vi "Known Targets.vi"() -> (3 "targets        project targetItem name              menu to use                    fpga sub                                           suffix info":T1(array[cluster])=[{"name"="My Computer", "owner"=TRUE, "none"=FALSE, "one"=FALSE, "auto"=FALSE, "choose"=FALSE, "opt#"=FALSE, "ipaddr"=FALSE, "[loc,]mod"=FALSE, "TSname"=""}, {"name"="Networked Computer/Device", "owner"=FALSE, "none"=TRUE, "one"=FALSE, "auto"=FALSE, "choose"=FALSE, "opt#"=TRUE, "ipaddr"=TRUE, "[loc,]mod"=FALSE, "TSname"="CPU"}, {"name"="RT Desktop Target", "owner"=FALSE, "none"=TRUE, "one"=FALSE, "auto"=FALSE, "choose"=FALSE, "opt#"=TRUE, "ipaddr"=TRUE, "[loc,]mod"=FALSE, "TSname"="RT cpu"}, {"name"="RT ELVIS RIO Target", "owner"=FALSE, "none"=TRUE, "one"=TRUE, "auto"=FALSE, "choose"=FALSE, "opt#"=TRUE, "ipaddr"=TRUE, "[loc,]mod"=FALSE, "TSname"="RT ELVIS"}, {"name"="RT myRIO Target", "owner"=FALSE, "none"=TRUE, "one"=TRUE, "auto"=FALSE, "choose"=FALSE, "opt#"=TRUE, "ipaddr"=TRUE, "[loc,]mod"=FALSE, "TSname"="RT myRIO"}, {"name"="RT CompactRIO Target", "owner"=FALSE, "none"=TRUE, "one"=TRUE, "auto"=FALSE, "choose"=FALSE, "opt#"=TRUE, "ipaddr"=TRUE, "[loc,]mod"=FALSE, "TSname"="RT cRIO"}, {"name"="RT Single-Board RIO Target", "owner"=FALSE, "none"=TRUE, "one"=TRUE, "auto"=FALSE, "choose"=FALSE, "opt#"=TRUE, "ipaddr"=TRUE, "[loc,]mod"=FALSE, "TSname"="RT sbRIO"}, {"name"="RT roboRIO Target", "owner"=FALSE, "none"=TRUE, "one"=TRUE, "auto"=FALSE, "choose"=FALSE, "opt#"=TRUE, "ipaddr"=TRUE, "[loc,]mod"=FALSE, "TSname"="RT roboRIO"}, {"name"="Ethernet RIO Target", "owner"=FALSE, "none"=TRUE, "one"=TRUE, "auto"=FALSE, "choose"=FALSE, "opt#"=TRUE, "ipaddr"=TRUE, "[loc,]mod"=FALSE, "TSname"="RT netRIO"}, {"name"="RT FlexRIO", "owner"=FALSE, "none"=TRUE, "one"=FALSE, "auto"=TRUE, "choose"=FALSE, "opt#"=TRUE, "ipaddr"=TRUE, "[loc,]mod"=FALSE, "TSname"="RT flexRIO"}, {"name"="RT PXI Target", "owner"=FALSE, "none"=FALSE, "one"=FALSE, "auto"=FALSE, "choose"=TRUE, "opt#"=FALSE, "ipaddr"=FALSE, "[loc,]mod"=FALSE, "TSname"="RT PXI"}, {"name"="FPGA Target", "owner"=FALSE, "none"=FALSE, "one"=FALSE, "auto"=FALSE, "choose"=FALSE, "opt#"=TRUE, "ipaddr"=FALSE, "[loc,]mod"=TRUE, "TSname"="FPGA"}])   [LabVIEW 2020, in "NI_TargetHelper.lvlib"]
uses:
  <vilib>/TargetSupport/NI_TargetHelper/NI_TargetHelper.lvlib
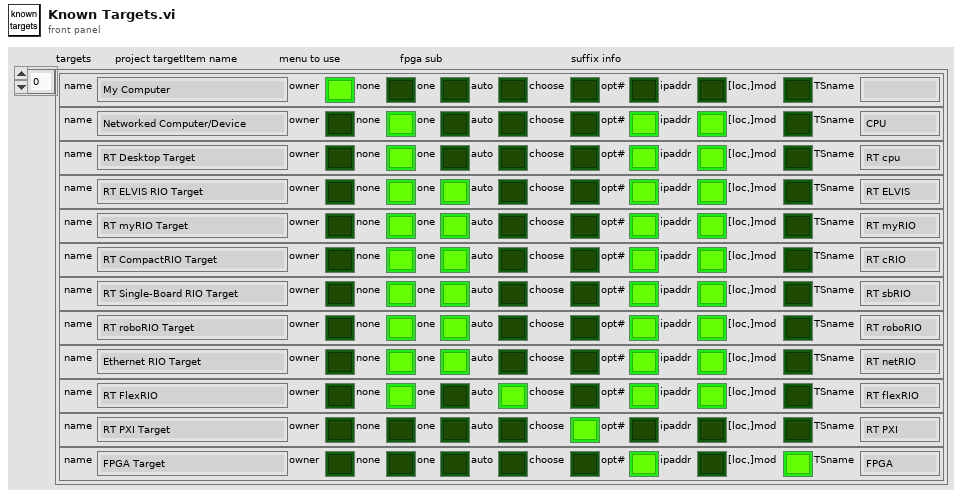
[diagram p1: front panel]
types:
  T1 = cluster{"name":string, "owner":bool, "none":bool, "one":bool, "auto":bool, "choose":bool, "opt#":bool, "ipaddr":bool, "[loc,]mod":bool, "TSname":string}[]
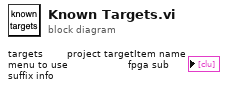
[diagram p0: block diagram]
diagram:
